vi "CLD1015_setpoint.vi"(7 "steps":u64, 8 "error CLD1015":errorcluster, 9 "stop":dbl, 10 "start":dbl, 11 "CLD1015 VISA":refnum<visa-resource-name>) -> (0 "error out":errorcluster, 1 "signal":dbl[](array[numeric]), 2 "current":dbl[](array[numeric]), 3 "CLD1015 VISA":refnum<visa-resource-name>, 5 "XY Graph":cluster{"X":dbl, "Y":dbl}[](graph))   [LabVIEW 2021]
uses:
  <vilib>/DAQmx/write.llb/DAQmx Write (Analog DBL 1Chan 1Samp).vi
  <vilib>/DAQmx/read.llb/DAQmx Read (Analog 1D DBL 1Chan NSamp).vi
  <vilib>/Analysis/baseanly.llb/Mean (DBL).vi
  <vilib>/DAQmx/create/channels.llb/DAQmx Create Channel (AI-Voltage-Basic).vi
  <vilib>/DAQmx/create/channels.llb/DAQmx Create Channel (AO-Voltage-Basic).vi
  <vilib>/DAQmx/miscellaneous.llb/DAQmx Fill In Error Info.vi
  <resource>/objmgr/daqmx.rc
  <vilib>/Analysis/NI_AALBase.lvlib
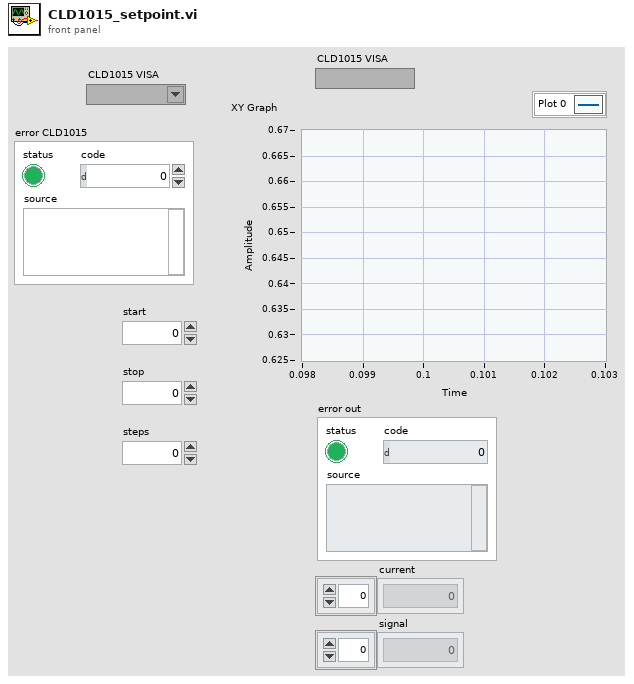
[diagram p1: front panel]
types:
  T1 = cluster{"output task":refnum<k21>, "input task":refnum<k21>, "error output":errorcluster, "error input":errorcluster, "CLD1015 VISA":refnum<visa-resource-name>, "error CLD1015":errorcluster}
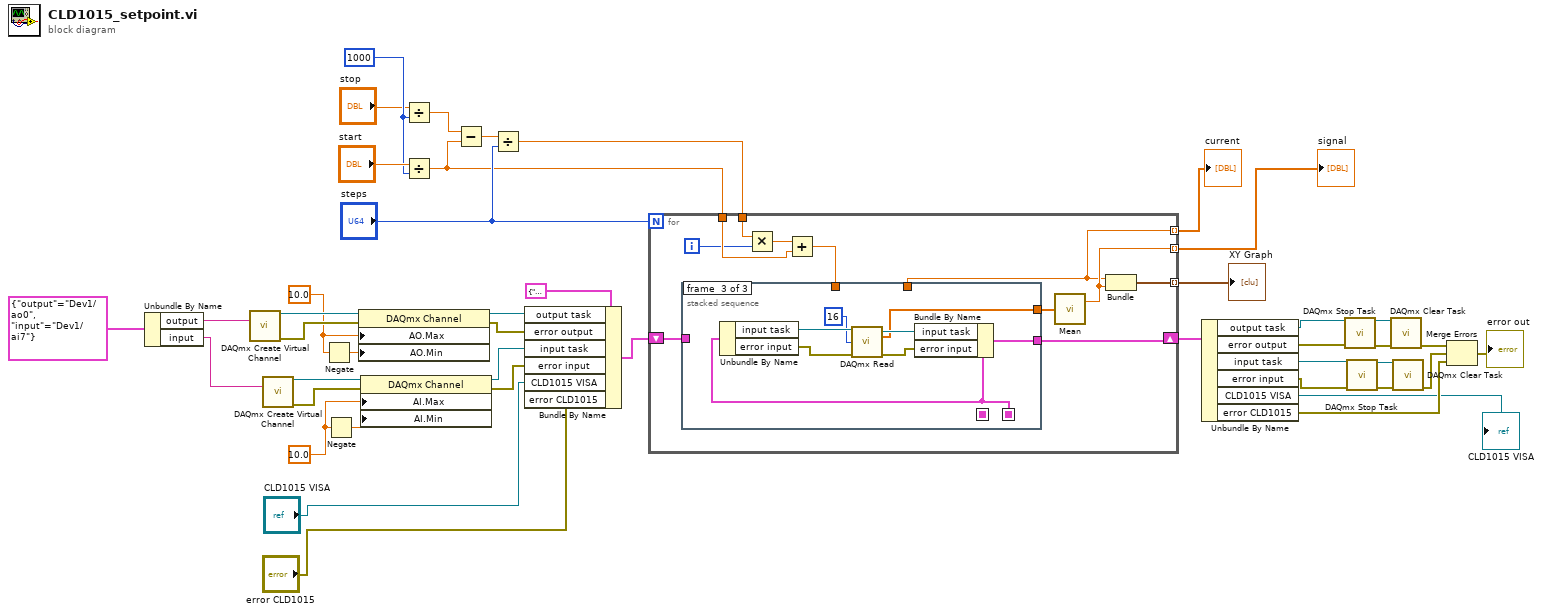
[diagram p0: block diagram]
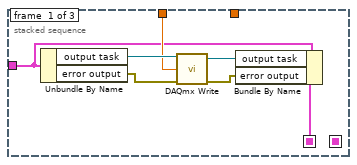
[diagram p2: hidden frame]
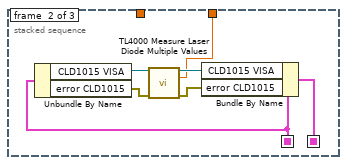
[diagram p3: hidden frame]
diagram:
  w11 = 1000
  w31 = 10.0
  w35 = 10.0
  n1 = Unbundle By Name(cluster{"output":tag, "input":tag} {"output"="Dev1/ao0", "input"="Dev1/ai7"}) -> ("output"=w44:tag, "input"=w42:tag)
  n2 = call-poly <vilib>:"DAQmx Create Virtual Channel.vi"("physical channels"=w44) -> ("task out"=w38:refnum<k21>, "error out"=w37:errorcluster)  [unwired: 13 in]
  n3 = call-poly <vilib>:"DAQmx Create Virtual Channel.vi"("physical channels"=w42) -> ("task out"=w29:refnum<k21>, "error out"=w30:errorcluster)  [unwired: 13 in]
  n4 = Negate(x=w35) -> (-x=w36:dbl)
  n5 = Negate(x=w31) -> (-x=w32:dbl)
  n6 = property class="DAQmx Channel"(reference=w38, error in=w37, "AO.Max"=w35, "AO.Min"=w36) -> (reference out=w34:refnum<k21>, error out=w33:errorcluster)
  n7 = property class="DAQmx Channel"(reference=w29, error in=w30, "AI.Max"=w31, "AI.Min"=w32) -> (reference out=w28:refnum<k21>, error out=w27:errorcluster)
  n8 = Divide(x="stop", y=w11) -> (x/y=w8:dbl)
  n9 = Divide(x="start", y=w11) -> (x/y=w10:dbl)
  n10 = Subtract(x=w8, y=w10) -> (x-y=w40:dbl)
  n11 = Divide(x=w40, y="steps") -> (x/y=w25:dbl)
  n12 = Bundle By Name(cluster=T1 {"output task"="", "input task"="", "error output"={"status"=FALSE, "code"=0, "source"=""}, "error input"={"status"=FALSE, "code"=0, "source"=""}, "CLD1015 VISA"="", "error CLD1015"={"status"=FALSE, "code"=0, "source"=""}}, "output task"=w34, "error output"=w33, "input task"=w28, "error input"=w27, "CLD1015 VISA"="CLD1015 VISA", "error CLD1015"="error CLD1015") -> (w26:T1)
  n13 = for {
    N: "steps" -> [_]
    shift-right: [w49] -> w24
    shift-left: w26 -> [w50]
    tunnel: w10 -> [w55]
    tunnel: w25 -> [w54]
    tunnel: [w47] -> w13 mode=indexing
    tunnel: [w46] -> w1 mode=indexing
    tunnel: [w45] -> w2 mode=indexing
    i -> [w53]
    n14 = Multiply(x=w54, y=w53) -> (x*y=w52:dbl)
    n15 = Add(x=w52, y=w55) -> (x+y=w51:dbl)
    n16 = stacked-sequence {
      seq-local: [w56 _ _] -> [_ w69 _]
      seq-local: [_ w68 _] -> [_ _ w70]
      tunnel: w51 -> [w60 _ _]
      tunnel: w50 -> [w59 _ _]
      tunnel: [_ _ w73] -> w49
      tunnel: [_ _ w71] -> w48
      tunnel: [_ w63 _] -> w45
      frame #0 {
        n17 = Unbundle By Name(w59) -> ("output task"=w62:refnum<k21>, "error output"=w61:errorcluster)
        n18 = call-poly <vilib>:"DAQmx Write.vi"("task/channels in"=w62, "data"=w60, "error in"=w61) -> ("task out"=w57:refnum<k21>, "error out"=w58:errorcluster)  [unwired: 10 in, 1 out]
        n19 = Bundle By Name(cluster=w59, "output task"=w57, "error output"=w58) -> (w56:T1)
      }
      frame #1 {
        n20 = Unbundle By Name(w69) -> ("CLD1015 VISA"=w67:refnum<visa-resource-name>, "error CLD1015"=w66:errorcluster)
        n21 = call <instrlib>:"TL4000 Measure Laser Diode Multiple Values.vi"("instrument handle"=w67, "error in (no error)"=w66) -> ("instrument handle out"=w65:refnum<visa-resource-name>, "Laser Current"=w63:dbl, "error out"=w64:errorcluster)  [unwired: 5 in, 6 out]
        n22 = Bundle By Name(cluster=w69, "CLD1015 VISA"=w65, "error CLD1015"=w64) -> (w68:T1)
      }
      frame #2 {
        n23 = Unbundle By Name(w70) -> ("input task"=w77:refnum<k21>, "error input"=w76:errorcluster)
        n24 = call-poly <vilib>:"DAQmx Read.vi"("task/channels in"=w77, "number of samples per channel"=16, "error in"=w76) -> ("task out"=w74:refnum<k21>, "data"=w71:dbl[], "error out"=w75:errorcluster)  [unwired: 10 in]
        n25 = Bundle By Name(cluster=w70, "input task"=w74, "error input"=w75) -> (w73:T1)
      }
    }
    n26 = call-poly <vilib>:"Mean.vi"("X"=w48) -> ("mean"=w46:dbl)  [unwired: 1 out]
    n27 = Bundle("Laser Current"=w45, "mean"=w46) -> (w47:cluster{"Laser Current":dbl, "mean":dbl})  [unwired: 1 in]
  }
  "XY Graph" <- w13
  "current" <- w2
  "signal" <- w1
  n28 = Unbundle By Name(w24) -> ("output task"=w19:refnum<k21>, "error output"=w18:errorcluster, "input task"=w17:refnum<k21>, "error input"=w16:errorcluster, "CLD1015 VISA"=→"CLD1015 VISA":refnum<visa-resource-name>, "error CLD1015"=w4:errorcluster)
  n29 = call <vilib>:"DAQmx Stop Task.vi"("task/channels in"=w19, "error in"=w18) -> ("task out"=w23:refnum<k21>, "error out"=w22:errorcluster)  [unwired: 12 in]
  n30 = call <vilib>:"DAQmx Stop Task.vi"("task/channels in"=w17, "error in"=w16) -> ("task out"=w20:refnum<k21>, "error out"=w21:errorcluster)  [unwired: 12 in]
  n31 = call <vilib>:"DAQmx Clear Task.vi"("task in"=w23, "error in"=w22) -> ("error out"=w15:errorcluster)  [unwired: 13 in]
  n32 = call <vilib>:"DAQmx Clear Task.vi"("task in"=w20, "error in"=w21) -> ("error out"=w14:errorcluster)  [unwired: 13 in]
  n33 = Merge Errors(w15, w14, w4) -> (→"error out":errorcluster)
